vi "UA_XML_stringtype.vi"(11 "XML String":string) -> (3 "XML Data":T1[](array[typedef]))   [LabVIEW 2013]
uses:
  UA_XML Data.ctl
  UA_RowType.ctl
panel:
  # "datatype=\"boolean\" initialValue=\"TRUE\"></item>"
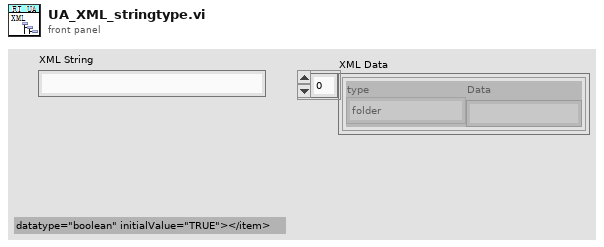
[diagram p1: front panel]
types:
  T1 = typedef "UA_XML Data.ctl" = cluster{"type":T2, "Data":string}
  T2 = typedef "UA_RowType.ctl" = enum16{"none", "folder", "item", "property", "folder end", "item end"}
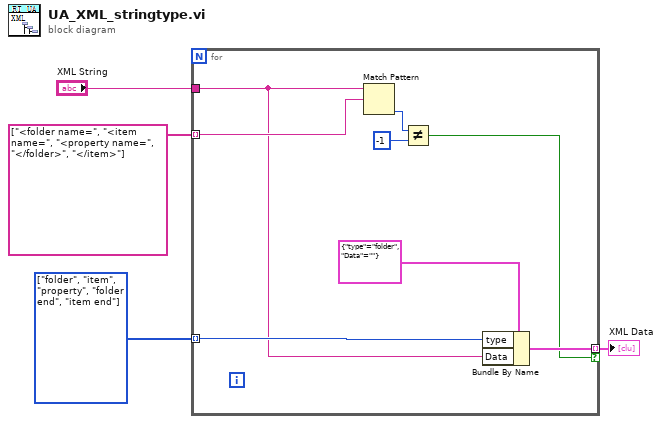
[diagram p0: block diagram]
diagram:
  w2 = T2[] [enum."folder", enum."item", enum."property", enum."folder end", enum."item end"] items=["none", "folder", "item", "property", "folder end", "item end"]
  n1 = for {
    tunnel: "XML String" -> [w5]
    tunnel: string[] ["<folder name=", "<item name=", "<property name=", "</folder>", "</item>"] ("start string") -> [w8] mode=indexing
    tunnel: w2 -> [w9] mode=indexing
    tunnel: [w7] -> w1 mode=indexing if=w6
    n2 = Match Pattern(string=w5, regular expression=w8) -> (offset past match=w12:i32)  [unwired: 1 in, 3 out]
    n3 = Not Equal?(x=w12, y=-1) -> (x != y?=w6:bool)
    n4 = Bundle By Name(cluster=T1 {"type"=enum."folder", "Data"=""} ("XML Data"), "type"=w9, "Data"=w5) -> (w7:T1)
  }
  "XML Data" <- w1
